vi "Set Trigger Source.vi"(8 "error in":errorcluster, 10 "Trigger Source":string(combo), 11 "VISA resource name in":refnum<visa-resource-name>) -> (0 "error out":errorcluster, 3 "VISA resource name out":refnum<visa-resource-name>)   [LabVIEW 2021, in "Keysight U1282A.lvlib"]
doc: "El comando definir la fuente de disparo (TRIG:SOUR) se utiliza para definir o salir del modo trigger hold o auto hold."
uses:
  Keysight U1282A.lvlib
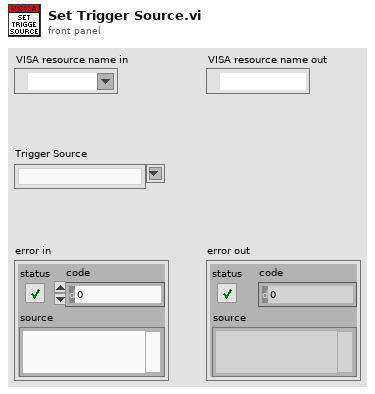
[diagram p1: front panel]
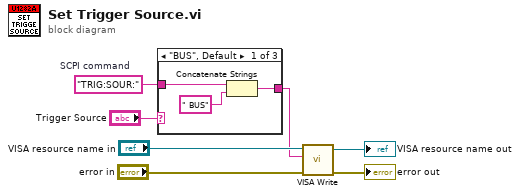
[diagram p0: block diagram]
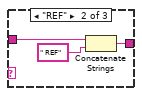
[diagram p2: hidden frame]
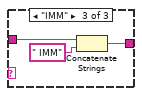
[diagram p3: hidden frame]
diagram:
  w6 = "TRIG:SOUR:"  # SCPI command
  n1 = case shown="\"BUS\", Default" "Trigger Source" {
    tunnel: w6 -> [w8 w12 w15]
    tunnel: [w9 w11 w14] -> w3
    frame "BUS", Default {
      n2 = Concatenate Strings(w8, " BUS") -> (w9:string)
    }
    frame "REF" {
      n3 = Concatenate Strings(w12, " REF") -> (w11:string)
    }
    frame "IMM" {
      n4 = Concatenate Strings(w15, " IMM") -> (w14:string)
    }
  }
  n5 = call "VISA Write.vi"("error in"="error in", "SCPI command"=w3, "VISA resource in"="VISA resource name in") -> ("error out"=→"error out":errorcluster, "VISA resource out"=→"VISA resource name out":refnum<visa-resource-name>)  [unwired: 6 in, 1 out]
